vi "WPI_IMU_IMUReset.vi"(3 "AHRS Reset In":dbl, 4 "Reset?":bool, 5 "Absolute Angle":dbl(slide) scale=-180.0..180.0) -> (0 "AHRS Reset Out":dbl, 2 "Converted Output":dbl(slide) scale=-180.0..180.0)   [LabVIEW 2015, in "FRC ADI MXP IMU.lvlib"]
uses:
  FRC ADI MXP IMU.lvlib
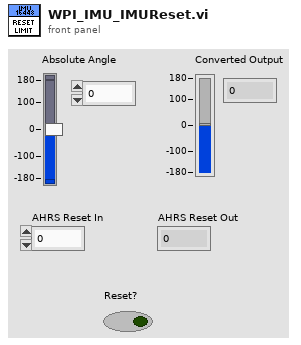
[diagram p1: front panel]
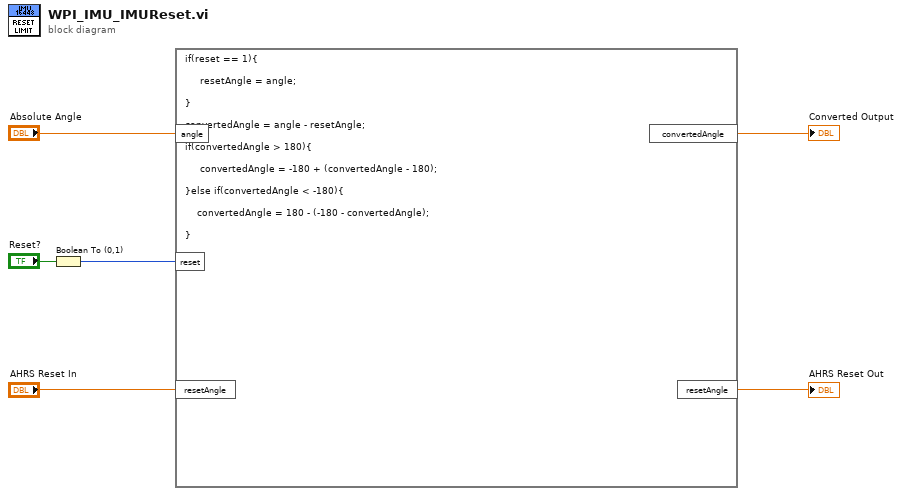
[diagram p0: block diagram]
diagram:
  n1 = Boolean To (0,1)(Boolean="Reset?") -> (0, 1=w2:i16)
  n2 = formula code="if(reset == 1){\n\t\t\t\n\t\t\t  resetAngle = angle;\n\n}\n\t\t\nconvertedAngle = angle - resetAngle;\n\t\t\nif(convertedAngle > 180){\n\t\t\t\n\t\t\t  convertedAngle = -180 + (convertedAngle - 180);\n\t\t\t\n}else if(convertedAngle < -180){\n\t\t\t\n\t\t  convertedAngle = 180 - (-180 - convertedAngle);\n\t\t\t\n}"("angle"="Absolute Angle", "reset"=w2, "resetAngle"="AHRS Reset In") -> ("convertedAngle"=→"Converted Output":dbl, "resetAngle"=→"AHRS Reset Out":dbl)
